vi "123.vi"() -> ()   [LabVIEW 2012]
uses:
  Control 1.ctl
  <vilib>/vision/NI_Vision_Development_Module.lvlib
panel:
  out "Frame Data":T1
  out "Number of Frames":u32
  in  "AVI Path":path
  out "2D Color value array":T2
  out "Image Pixels (U32)":u32[][](array[numeric])
  out "Path":path
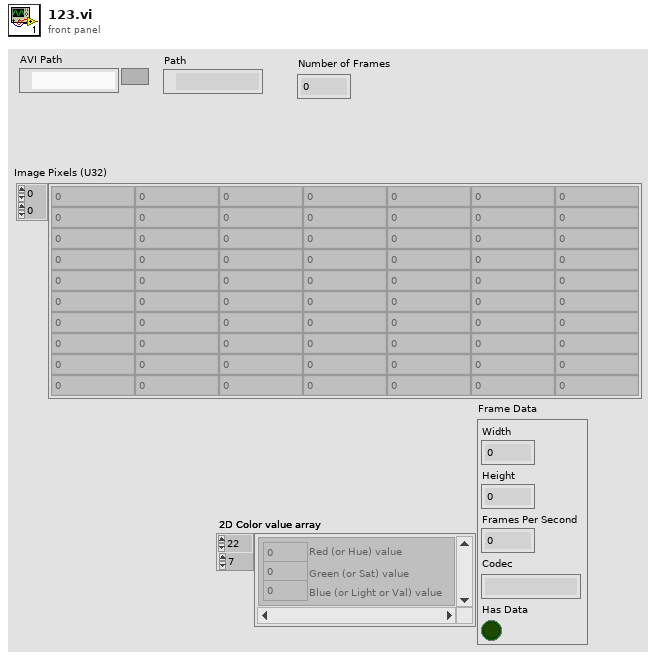
[diagram p1: front panel]
types:
  T1 = cluster{"Width":u32, "Height":u32, "Frames Per Second":u32, "Codec":string, "Has Data":bool}
  T2 = typedef "Control 1.ctl" = cluster{"Red (or Hue) value":u8, "Green (or Sat) value":u8, "Blue (or Light or Val) value":u8}[][]
  T3 = typedef "IMAQ AVI2 Refnum.ctl" = refnum<k20>
  T4 = typedef "Image Type" = u32
  T5 = typedef "IMAQ Image.ctl" = refnum<image>
  T6 = cluster{"Red (or Hue) value":u8, "Green (or Sat) value":u8, "Blue (or Light or Val) value":u8}[][]
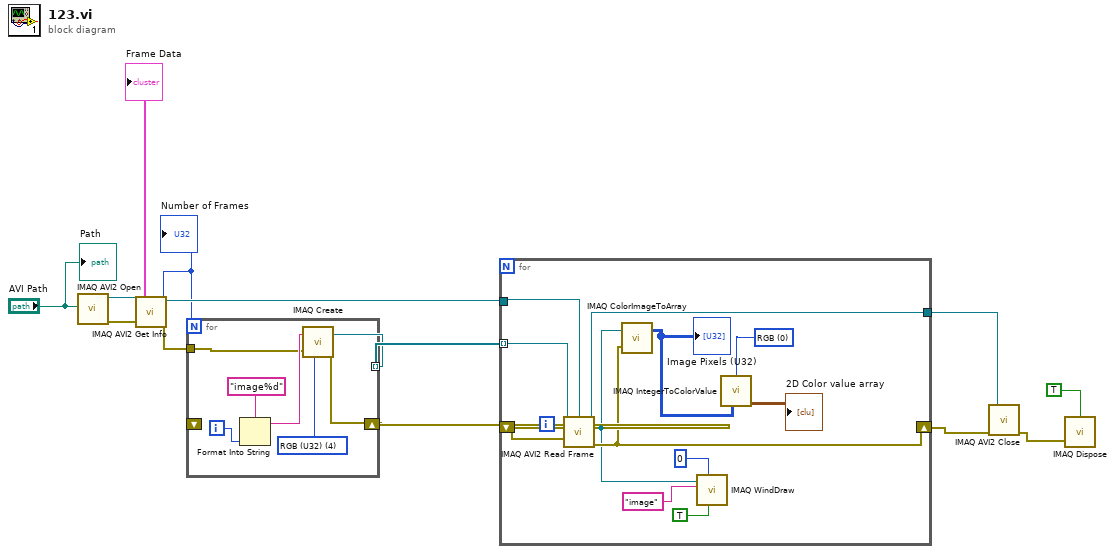
[diagram p0: block diagram]
diagram:
  n1 = call "IMAQ AVI2 Open"("AVI File Path"="AVI Path") -> ("error out"=w11:errorcluster, "AVI Refnum"=w12:T3)  [unwired: 9 in]
  n2 = call "IMAQ AVI2 Get Info"("error in (no error)"=w11, "AVI Refnum"=w12) -> ("error out"=w8:errorcluster, "Number of Frames"=w3:u32, "AVI Refnum (duplicate)"=w10:T3, "Frame Data"=→"Frame Data":T1)  [unwired: 5 in, 1 out]
  "Number of Frames" <- w3
  n3 = for {
    N: w3 -> [_]
    tunnel: [w17] -> w9 mode=indexing
    tunnel: w8 -> [w14]
    shift-right: [w16] -> w6
    shift-left: _ -> [_]
    i -> [w15]
    w18 = T4 4 items=["Grayscale (U8)", "Grayscale (I16)", "Grayscale (SGL)", "Complex (CSG)", "RGB (U32)", "HSL (U32)", "RGB (U64)", "Grayscale (U16)"]
    n4 = Format Into String(format string="image%d" ("Image Name"), w15) -> (resulting string=w20:string)  [unwired: 2 in, 1 out]
    n5 = call "IMAQ Create"("Image Name"=w20, "Image Type"=w18, "error in (no error)"=w14) -> ("New Image"=w17:T5, "error out"=w16:errorcluster)  [unwired: 2 in]
  }
  n6 = for {
    tunnel: w10 -> [w33]
    tunnel: w9 -> [w32] mode=indexing
    shift-right: [w26] -> w2
    shift-left: w6 -> [w28]
    tunnel: [w25] -> w4
    i -> [w27]
    w29 = u16 0 items=["RGB", "HSL", "HSV", "HSI"] ("Color Mode")
    n7 = call "IMAQ AVI2 Read Frame"("error in (no error)"=w28, "Frame Number"=w27, "Image"=w32, "AVI Refnum"=w33) -> ("error out"=w26:errorcluster, "Image Out"=w24:T5, "AVI Refnum (duplicate)"=w25:T3)  [unwired: 5 in]
    n8 = call "IMAQ ColorImageToArray"("Image"=w24, "error in (no error)"=w26) -> ("Image Pixels (U32)"=w31:u32[][])  [unwired: 2 in, 2 out]
    "Image Pixels (U32)" <- w31
    n9 = call "IMAQ WindDraw"("Resize to Image Size? (Y)"=TRUE, "Window Number (0...15)"=0, "Title"="image", "Image"=w24) -> ()  [unwired: 6 in, 2 out]
    n10 = call "IMAQ IntegerToColorValue"("2D U32 array"=w31, "Color Mode"=w29) -> ("2D Color value array"=→"2D Color value array":T6)  [unwired: 3 in, 3 out]
  }
  n11 = call "IMAQ AVI2 Close"("error in (no error)"=w2, "AVI Refnum"=w4) -> ("error out"=w5:errorcluster)  [unwired: 9 in]
  n12 = call "IMAQ Dispose"("All Images? (No)"=TRUE, "error in (no error)"=w5) -> ()  [unwired: 4 in, 1 out]
  "Path" <- "AVI Path"
